vi "Extract.vi"(8 "error in (no error)":errorcluster, 10 "AbstractData in":refnum<class "AbstractData.lvclass">, 11 "AbstractExtractor in":refnum<class "AbstractExtractor.lvclass">) -> (0 "error out":errorcluster, 3 "AbstractExtractor out":refnum<class "AbstractExtractor.lvclass">)   [LabVIEW 2014, in "AbstractExtractor.lvclass"]
uses:
  AbstractExtractor.lvclass
  Model/Data/AbstractData/AbstractData.lvclass
  Interfaces/Observable Actor/Observable Actor.lvclass
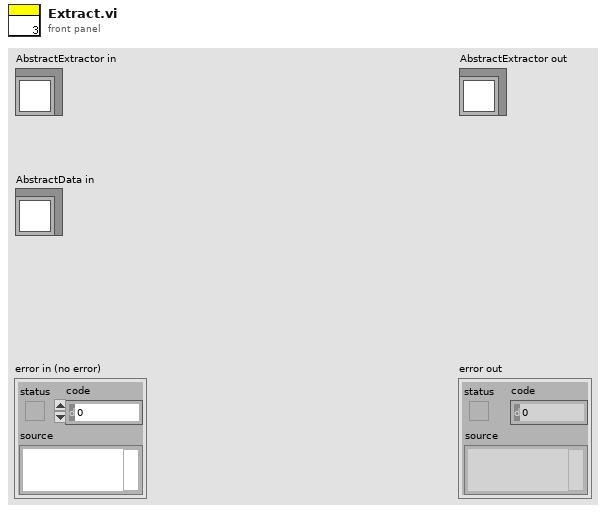
[diagram p1: front panel]
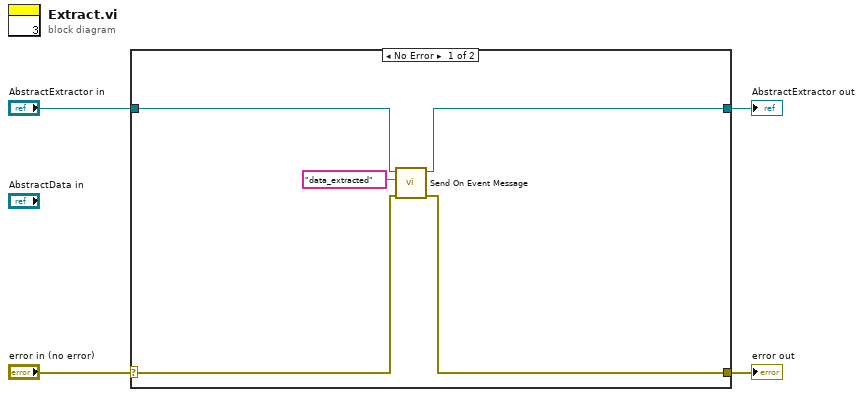
[diagram p0: block diagram]
diagram:
  n1 = case shown="No Error" "error in (no error)" {
    selector: "error in (no error)" -> [w6 w11]
    tunnel: [w5 w11] -> w3
    tunnel: [w8 w10] -> w1
    tunnel: "AbstractExtractor in" -> [w9 w10]
    frame No Error {
      n2 = call "Send On Event Message.vi"("error in (no error)"=w6, "Event"="data_extracted", "Observable Actor in"=w9) -> ("error out"=w5:errorcluster, "Observable Actor out"=w8:refnum<class "AbstractExtractor.lvclass">)  [unwired: 7 in]
    }
    frame Error {
    }
  }
  "error out" <- w3
  "AbstractExtractor out" <- w1
